vi "CreateFakeTestCase.vi"(8 "error in (no error)":errorcluster, 10 "Name":string) -> (0 "error out":errorcluster, 3 "FakeTestCase out":refnum<class "FakeTestCase.lvclass">)   [LabVIEW 2017, in "ResultTreeListenerTest.lvlib" / "Support.lvlib" / "FakeTestCase.lvclass"]
uses:
  FakeTestCase.lvclass
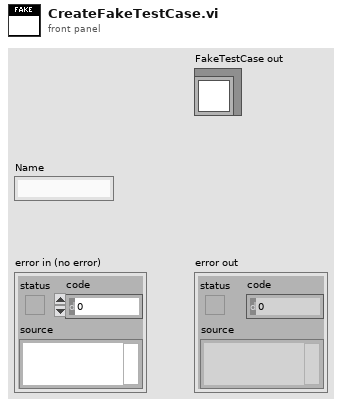
[diagram p1: front panel]
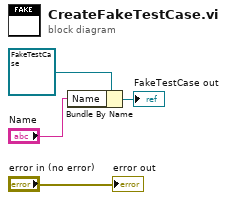
[diagram p0: block diagram]
diagram:
  n1 = Bundle By Name(cluster=refnum<class "FakeTestCase.lvclass"> refnum ("FakeTestCase in"), "Name"="Name") -> (→"FakeTestCase out":refnum<class "FakeTestCase.lvclass">)
  "error out" <- "error in (no error)"
